vi "Get Row and Colum - Single Pixel (SubVI).vi"(8 "Dim":u32=256, 9 "Current pixel base (row)":u32=256, 10 "Colum In":u32, 11 "Row In":u32) -> (0 "Last Pixel?":bool, 1 "Next pixel base (row)":u32, 2 "Colum Out":u32, 3 "Row Out":u32, 6 "Pixel":u32)   [LabVIEW 2017]
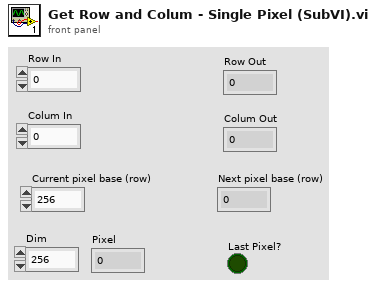
[diagram p1: front panel]
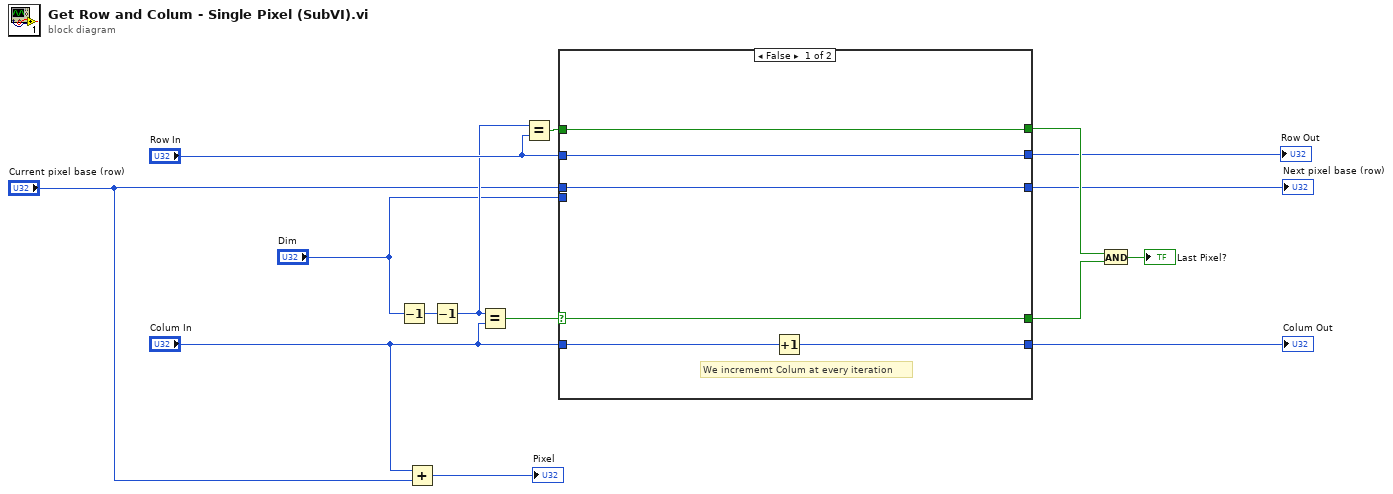
[diagram p0: block diagram]
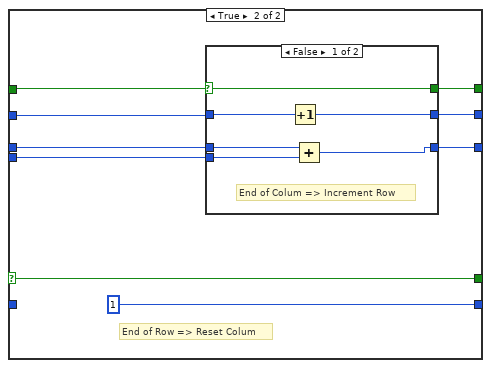
[diagram p2: hidden frame]
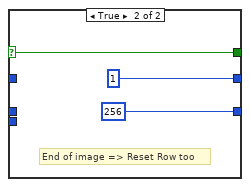
[diagram p3: hidden frame]
diagram:
  n1 = Decrement(x="Dim") -> (x-1=w5:u32)
  n2 = Add(x="Colum In", y="Current pixel base (row)") -> (x+y=→"Pixel":u32)
  n3 = Decrement(x=w5) -> (x-1=w4:u32)
  n4 = Equal?(x=w4, y="Colum In") -> (x = y?=w15:bool)
  n5 = Equal?(x=w4, y="Row In") -> (x = y?=w9:bool)
  n6 = case shown="False" w15 {
    selector: w15 -> [w19 w29]
    tunnel: [w21 u32 1] -> w14
    tunnel: "Colum In" -> [w20 _]
    tunnel: [w19 w29] -> w13
    tunnel: w9 -> [w17 w28]
    tunnel: "Row In" -> [w18 w25]
    tunnel: [w18 w27] -> w6
    tunnel: [w17 w26] -> w8
    tunnel: [w16 w24] -> w3
    tunnel: "Current pixel base (row)" -> [w16 w23]
    tunnel: "Dim" -> [_ w22]
    frame False {
      # "We incrememt Colum at every iteration"
      n7 = Increment(x=w20) -> (x+1=w21:u32)
    }
    frame True {
      # "End of Row => Reset Colum"
      n8 = case shown="False" w28 {
        selector: w28 -> [w34 w38]
        tunnel: [w35 u32 1] -> w27
        tunnel: w25 -> [w36 _]
        tunnel: [w34 w38] -> w26
        tunnel: [w32 u32 256] -> w24
        tunnel: w23 -> [w33 _]
        tunnel: w22 -> [w31 _]
        frame False {
          # "End of Colum => Increment Row"
          n9 = Increment(x=w36) -> (x+1=w35:u32)
          n10 = Add(x=w33, y=w31) -> (x+y=w32:u32)
        }
        frame True {
          # "End of image => Reset Row too"
        }
      }
    }
  }
  "Row Out" <- w6
  "Colum Out" <- w14
  "Next pixel base (row)" <- w3
  n11 = And(x=w8, y=w13) -> (x .and. y?=→"Last Pixel?":bool)
